vi "String IP To WebDAV Uri.vi"(7 "File Location":string="/files", 10 "IP In":string) -> (2 "WebDAV Uri Out":string)   [LabVIEW 2024]
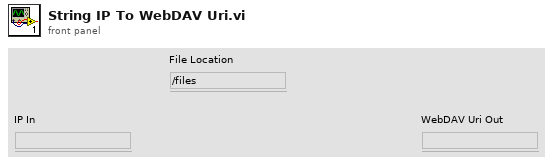
[diagram p1: front panel]
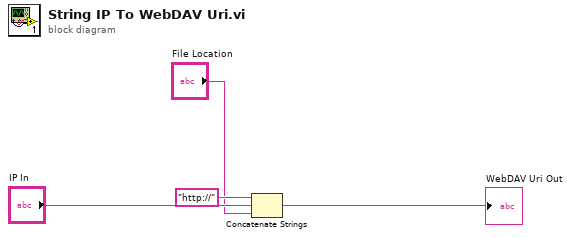
[diagram p0: block diagram]
diagram:
  n1 = Concatenate Strings("http://" ("string"), "IP In", "File Location") -> (→"WebDAV Uri Out":string)
